vi "LM call model function.vi"(7 "model function":T2, 8 "error in (no error)":errorcluster, 9 "output control":T1, 10 "X":dbl[](array[numeric]), 11 "a":dbl[](array[numeric])) -> (0 "error out":errorcluster, 1 "number of function evaluations":i32, 2 "f'(X,a)":dbl[][](array[numeric]), 3 "f(X)":dbl[](array[numeric]))   [LabVIEW 2010, in "NI_Gmath.lvlib"]
uses:
  NI_Gmath.lvlib
  LM model function.ctl
  LM model function reference.ctl
  LM_output select.ctl
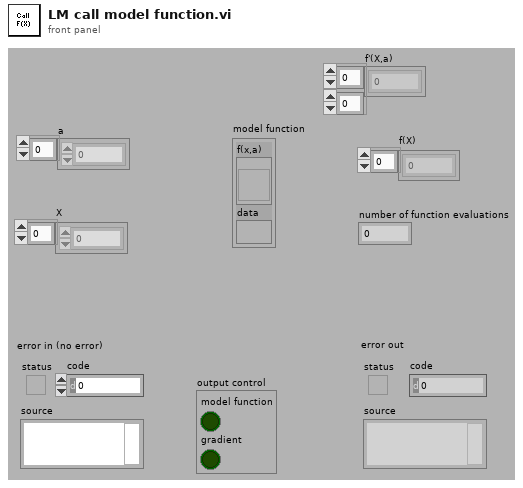
[diagram p1: front panel]
types:
  T1 = typedef "NI_Gmath.lvlib/LM_output select.ctl" = cluster{"model function":bool, "gradient":bool}
  T2 = typedef "NI_Gmath.lvlib/LM model function.ctl" = cluster{"f(x,a)":T3, "data":variant}
  T3 = typedef "NI_Gmath.lvlib/LM model function reference.ctl" = refnum<vi>
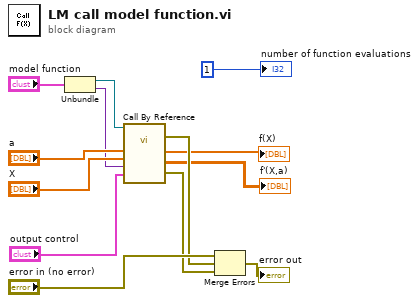
[diagram p0: block diagram]
diagram:
  n1 = Unbundle("model function") -> ("f(x,a)"=w2:T3, "data"=w1:variant)
  n2 = call-by-ref "?"(reference=w2, "output control"="output control", "data"=w1, "X"="X", "a"="a") -> (error out=w11:errorcluster, 0:"error out"=w9:errorcluster, "f'(X,a)"=→"f'(X,a)":dbl[][], "f(X,a)"=→"f(X)":dbl[])  [unwired: 1 in, 1 out]
  n3 = Merge Errors("error in (no error)", w11, w9) -> (→"error out":errorcluster)
  "number of function evaluations" <- 1
